vi "Test manual launch.vi"() -> ()   [LabVIEW 2021]
uses:
  <vilib>/Utility/LVLibp/NI_PackedLibraryUtility.lvlib
panel:
  out "error out":errorcluster
  out "data":string
  out "error out 2":errorcluster
  out "qualified names":string[](array[string])=["CIFTemplatePlugin.lvlibp:Energize.vi", "CIFTemplatePlugin.lvlibp:Launch.vi"]
  in  "Linux":path=path "/home/lvuser/natinst/bin/CIFTemplatePlugin.lvlibp"
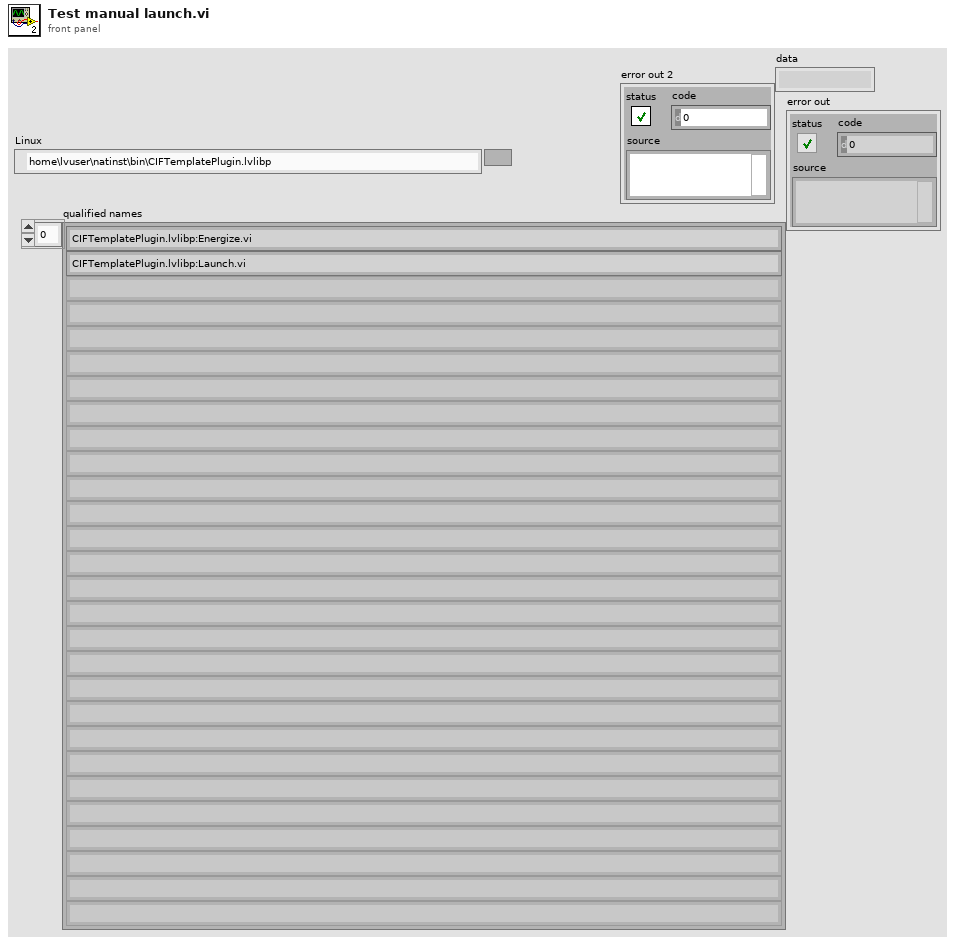
[diagram p1: front panel]
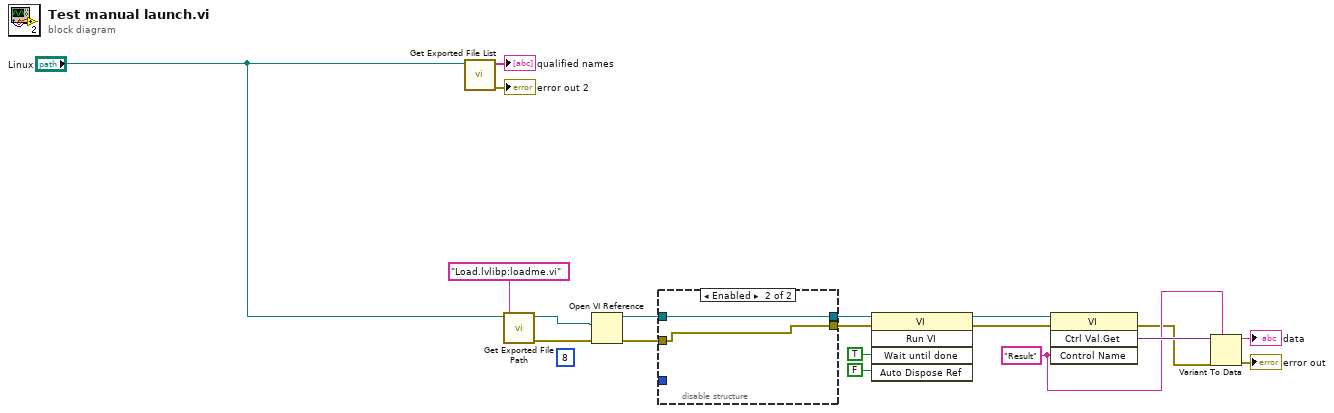
[diagram p0: block diagram]
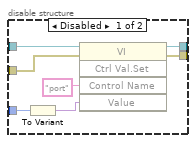
[diagram p2: hidden frame]
diagram:
  w4 = "Result" ("Control Name")
  (unwired) 8 ("options")
  n1 = call <vilib>:"Get Exported File List.vi"("packed library path"="Linux") -> ("error out"=→"error out 2":errorcluster, "qualified names"=→"qualified names":string[])  [unwired: 8 in, 1 out]
  n2 = call <vilib>:"Get Exported File Path.vi"("qualified name"="Load.lvlibp:loadme.vi", "packed library path"="Linux") -> ("error out"=w13:errorcluster, "path"=w12:path)  [unwired: 8 in]
  n3 = Open VI Reference(vi path=w12, error in (no error)=w13) -> (vi reference=w8:refnum<vi>, error out=w15:errorcluster)  [unwired: 4 in]
  n4 = disable-structure shown="Enabled" {
    disable-tunnel: _ -> [w26 _]
    disable-tunnel: [w23 w27] -> w9
    disable-tunnel: [w22 w28] -> w10
    disable-tunnel: w15 -> [w21 w27]
    disable-tunnel: w8 -> [w20 w28]
    frame Disabled {
      n5 = To Variant(anything=w26) -> (Variant=w25:variant)
      n6 = invoke class="VI" method="Ctrl Val.Set"(reference=w20, error in=w21, "Control Name"="port", "Value"=w25) -> (reference out=w22:refnum<vi>, error out=w23:errorcluster)  [unwired: 1 in, 3 out]
    }
    frame Enabled {
    }
  }
  n7 = invoke class="VI" method="Run VI"(reference=w10, error in=w9, "Wait until done"=TRUE ("Wait Until Done"), "Auto Dispose Ref"=FALSE ("Auto Dispose Reference")) -> (reference out=w7:refnum<vi>, error out=w6:errorcluster)  [unwired: 1 in, 3 out]
  n8 = invoke class="VI" method="Ctrl Val.Get"(reference=w7, error in=w6, "Control Name"=w4) -> (error out=w2:errorcluster, "Get Control Value Variant"=w5:variant)  [unwired: 1 in, 2 out]
  n9 = Variant To Data(error in=w2, type=w4, Variant=w5) -> (data=→"data":string, error out=→"error out":errorcluster)
